vi "SALICRUPythonFile(SubVI).vi"() -> (3 "SALICRU WRAPPER FILE":path)   [LabVIEW 2024]
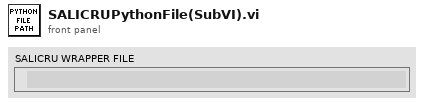
[diagram p1: front panel]
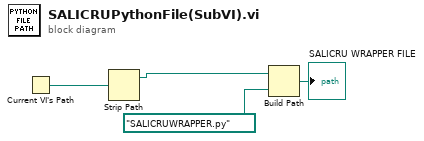
[diagram p0: block diagram]
diagram:
  n1 = Current VI's Path() -> (path=w1:path)
  n2 = Strip Path(path=w1) -> (stripped path=w2:path)  [unwired: 1 out]
  n3 = Build Path(base path=w2, name or relative path=path "SALICRUWRAPPER.py") -> (appended path=→"SALICRU WRAPPER FILE":path)
